vi "Create file and SetCellValuesInXLS.vi"() -> ()   [LabVIEW 2013]
uses:
  Sheet/Polymorphic VIs/Set Cell (String).vi
  Sheet/Polymorphic VIs/Set Cell (DBL).vi
panel:
  out "Last Row":i32
  out "Last Column":i32
  in  "File Name":path=path "C:/PhaeronGit/LVNPOI/Scratch/test.xls"
  # "These are zero-based."
  # "LabVIEW implementation of SetCellValuesInXLS.cs"
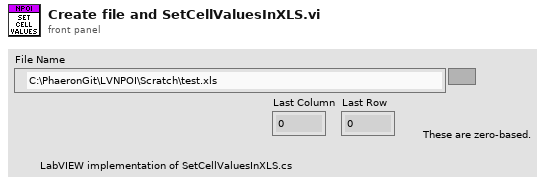
[diagram p1: front panel]
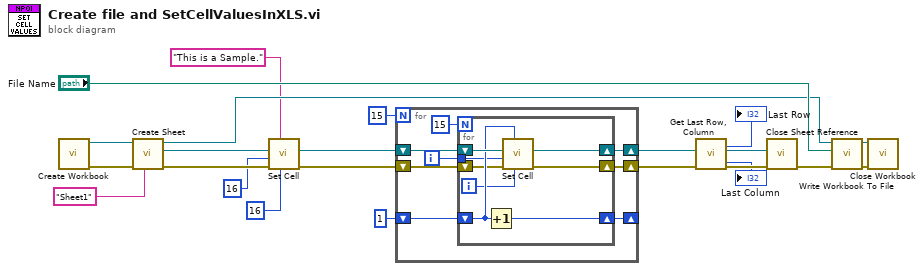
[diagram p0: block diagram]
diagram:
  n1 = call "Create Workbook.vi"() -> ("error out"=w19:errorcluster, "hssfworkbook"=w20:refnum<k24>)  [unwired: 10 in]
  n2 = call "Create Sheet.vi"("Sheet Name (Sheet1)"="Sheet1" ("sheetname"), "error in (no error)"=w19, "Workbook Reference"=w20) -> ("error out"=w14:errorcluster, "Sheet Reference"=w15:refnum<k24>, "Workbook Reference"=w18:refnum<k24>)  [unwired: 6 in]
  n3 = call-poly "Set Cell.vi"("Column"=16 ("column"), "Value"="This is a Sample." ("value"), "error in (no error)"=w14, "Row"=16 ("rownum"), "Sheet Reference"=w15) -> ("error out"=w10:errorcluster, "Sheet Reference out"=w11:refnum<k24>)  [unwired: 5 in]
  n4 = for {
    N: 15 -> [_]
    shift-right: [w25] -> w4
    shift-left: w11 -> [w28]
    shift-right: [w24] -> w6
    shift-left: w10 -> [w26]
    shift-right: [w30] -> _
    shift-left: 1 -> [w31]
    i -> [w27]
    n5 = for {
      N: 15 -> [_]
      shift-right: [w39] -> w30
      shift-left: w31 -> [w37]
      shift-right: [w32] -> w24
      shift-left: w26 -> [w33]
      tunnel: w27 -> [w36]
      shift-right: [w34] -> w25
      shift-left: w28 -> [w38]
      i -> [w35]
      n6 = Increment(x=w37) -> (x+1=w39:i32)
      n7 = call-poly "Set Cell.vi"("Column"=w35, "Value"=w37, "error in (no error)"=w33, "Row"=w36, "Sheet Reference"=w38) -> ("error out"=w32:errorcluster, "Sheet Reference out"=w34:refnum<k24>)  [unwired: 5 in]
    }
  }
  n8 = call "Get Last Row, Column.vi"("error in (no error)"=w6, "Sheet Reference"=w4) -> ("error out"=w5:errorcluster, "Sheet Reference out"=w3:refnum<k24>, "Last Column"=→"Last Column":i32, "Last Row"=→"Last Row":i32)  [unwired: 6 in]
  n9 = call "Close Sheet Reference.vi"("error in (no error)"=w5, "Sheet Reference"=w3) -> ("error out"=w7:errorcluster)  [unwired: 9 in]
  n10 = call "Write Workbook To File.vi"("error in (no error)"=w7, "File Name"="File Name", "Workbook Reference"=w18) -> ("error out"=w8:errorcluster, "Workbook Reference Out"=w9:refnum<k24>)  [unwired: 7 in]
  n11 = call "Close Workbook.vi"("error in (no error)"=w8, "Workbook Reference"=w9) -> ()  [unwired: 9 in, 1 out]
